vi "Item Not Found and Invalid Reference.vi"(10 "found?":bool, 11 "item reference":T1=18446744073709551615 format="%.0x") -> (3 "no item found":bool)   [LabVIEW 2020, in "Scripting.lvclass"]
uses:
  Scripting.lvclass
  <vilib>/NI VeriStand/Custom Device API/Custom Device Item Ref.ctl
  <vilib>/NI VeriStand/Custom Device API/Custom Device API.lvlib
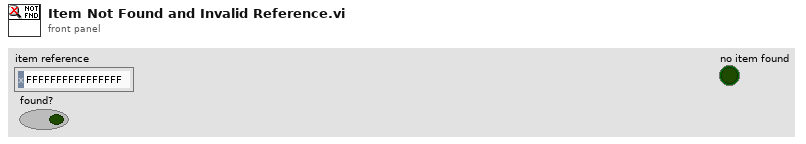
[diagram p1: front panel]
types:
  T1 = typedef "Custom Device API.lvlib/Custom Device Item Ref.ctl" = u64
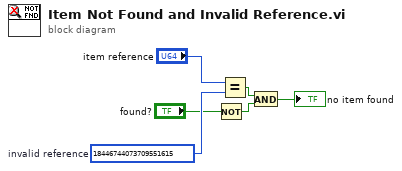
[diagram p0: block diagram]
diagram:
  w4 = T1 18446744073709551615  # invalid reference
  n1 = Not(x="found?") -> (.not. x?=w6:bool)
  n2 = Equal?(x="item reference", y=w4) -> (x = y?=w5:bool)
  n3 = And(x=w5, y=w6) -> (x .and. y?=→"no item found":bool)
